vi "mqttTCPIPserver.vi"(0 "mqtt.lvclass":refnum<class "mqtt.lvclass">, 11 "error in (no error)":errorcluster) -> (4 "mqtt.lvclass 2":refnum<class "mqtt.lvclass">, 15 "error out":errorcluster)   [LabVIEW 2022 SP3, in "mqtt.lvclass"]
uses:
  mqtt.lvclass
  mqttTXqueue/mqttTXdataQueueFunction.ctl
  mqtt.lvclass/mqtt.ctl
  mqttTypedef/mqttRXdataCluster.ctl
  mqttTypedef/mqttFixedHeaderResponse.ctl
  mqttTypedef/mqttQOSlevel.ctl
  mqttTypedef/mqttMessageType.ctl
  mqttTXqueue/mqttRXsubscriptionEventFunction.ctl
  mqttTXqueue/mqttRXsubscriptionEventData.ctl
panel:
  out "rxCount":i32
  out "rxTelegram":u8[](array[numeric]) format="%02x"
  out "txError":errorcluster
  out "txTelegram":u8[](array[numeric]) format="%02x"
  out "payloadError":errorcluster
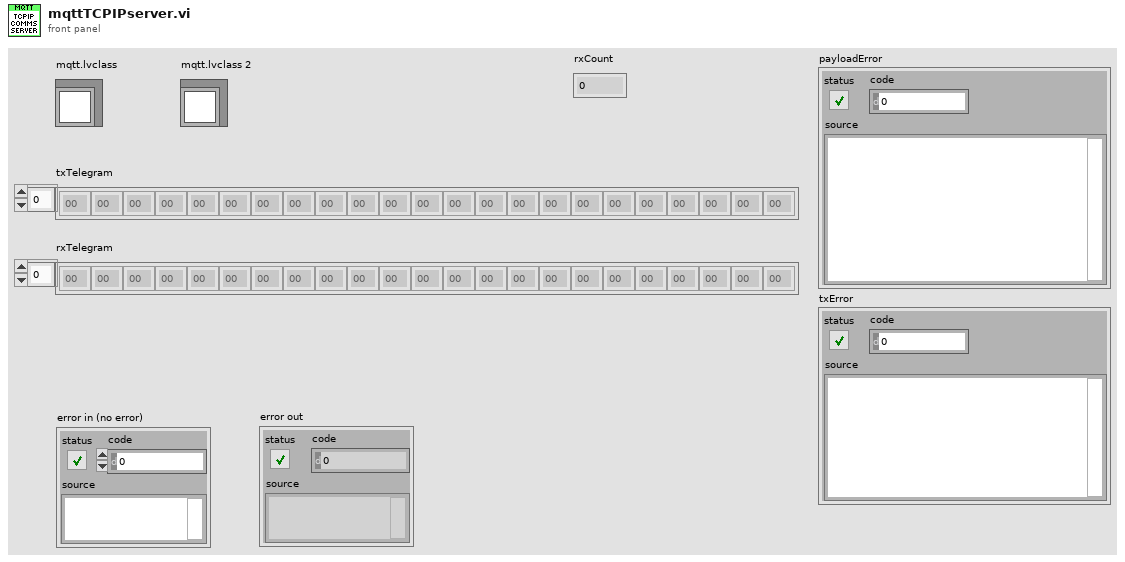
[diagram p1: front panel]
types:
  T1 = typedef "mqttTXdataQueueFunction.ctl" = enum16{"init", "deinit", "getQueue", "enqueue"}
  T2 = typedef "mqttRXdataCluster.ctl" = cluster{"fixedHdr":T3, "payload":u8[]}
  T3 = typedef "mqttFixedHeaderResponse.ctl" = cluster{"retain":bool, "qos":T4, "duplicate":bool, "response":T5}
  T4 = typedef "mqttQOSlevel.ctl" = enum8{"At most once", "At least once", "Exactly once", "Reserved"}
  T5 = typedef "mqttMessageType.ctl" = enum32{"Reserved", "CONNECT", "CONNACK", "PUBLISH", "PUBACK", "PUBREC", "PUBREL", "PUBCOMP", "SUBSCRIBE", "SUBACK", "UNSUBSCRIBE", "UNSUBACK", "PINGREQ", "PINGRESP", "DISCONNECT", "Reserved2"}
  T6 = typedef "mqttRXsubscriptionEventData.ctl" = cluster{"topic":string, "value":string, "messageID":u16}
  T7 = typedef "mqttRXsubscriptionEventFunction.ctl" = enum16{"init", "deinit", "getEventRef", "event"}
  T8 = typedef "mqttBroker.ctl" = cluster{"address":string, "port":u16, "connTimeout":i32, "writeTimeout":i32, "readTimeout":i32, "subTimeout":i32}
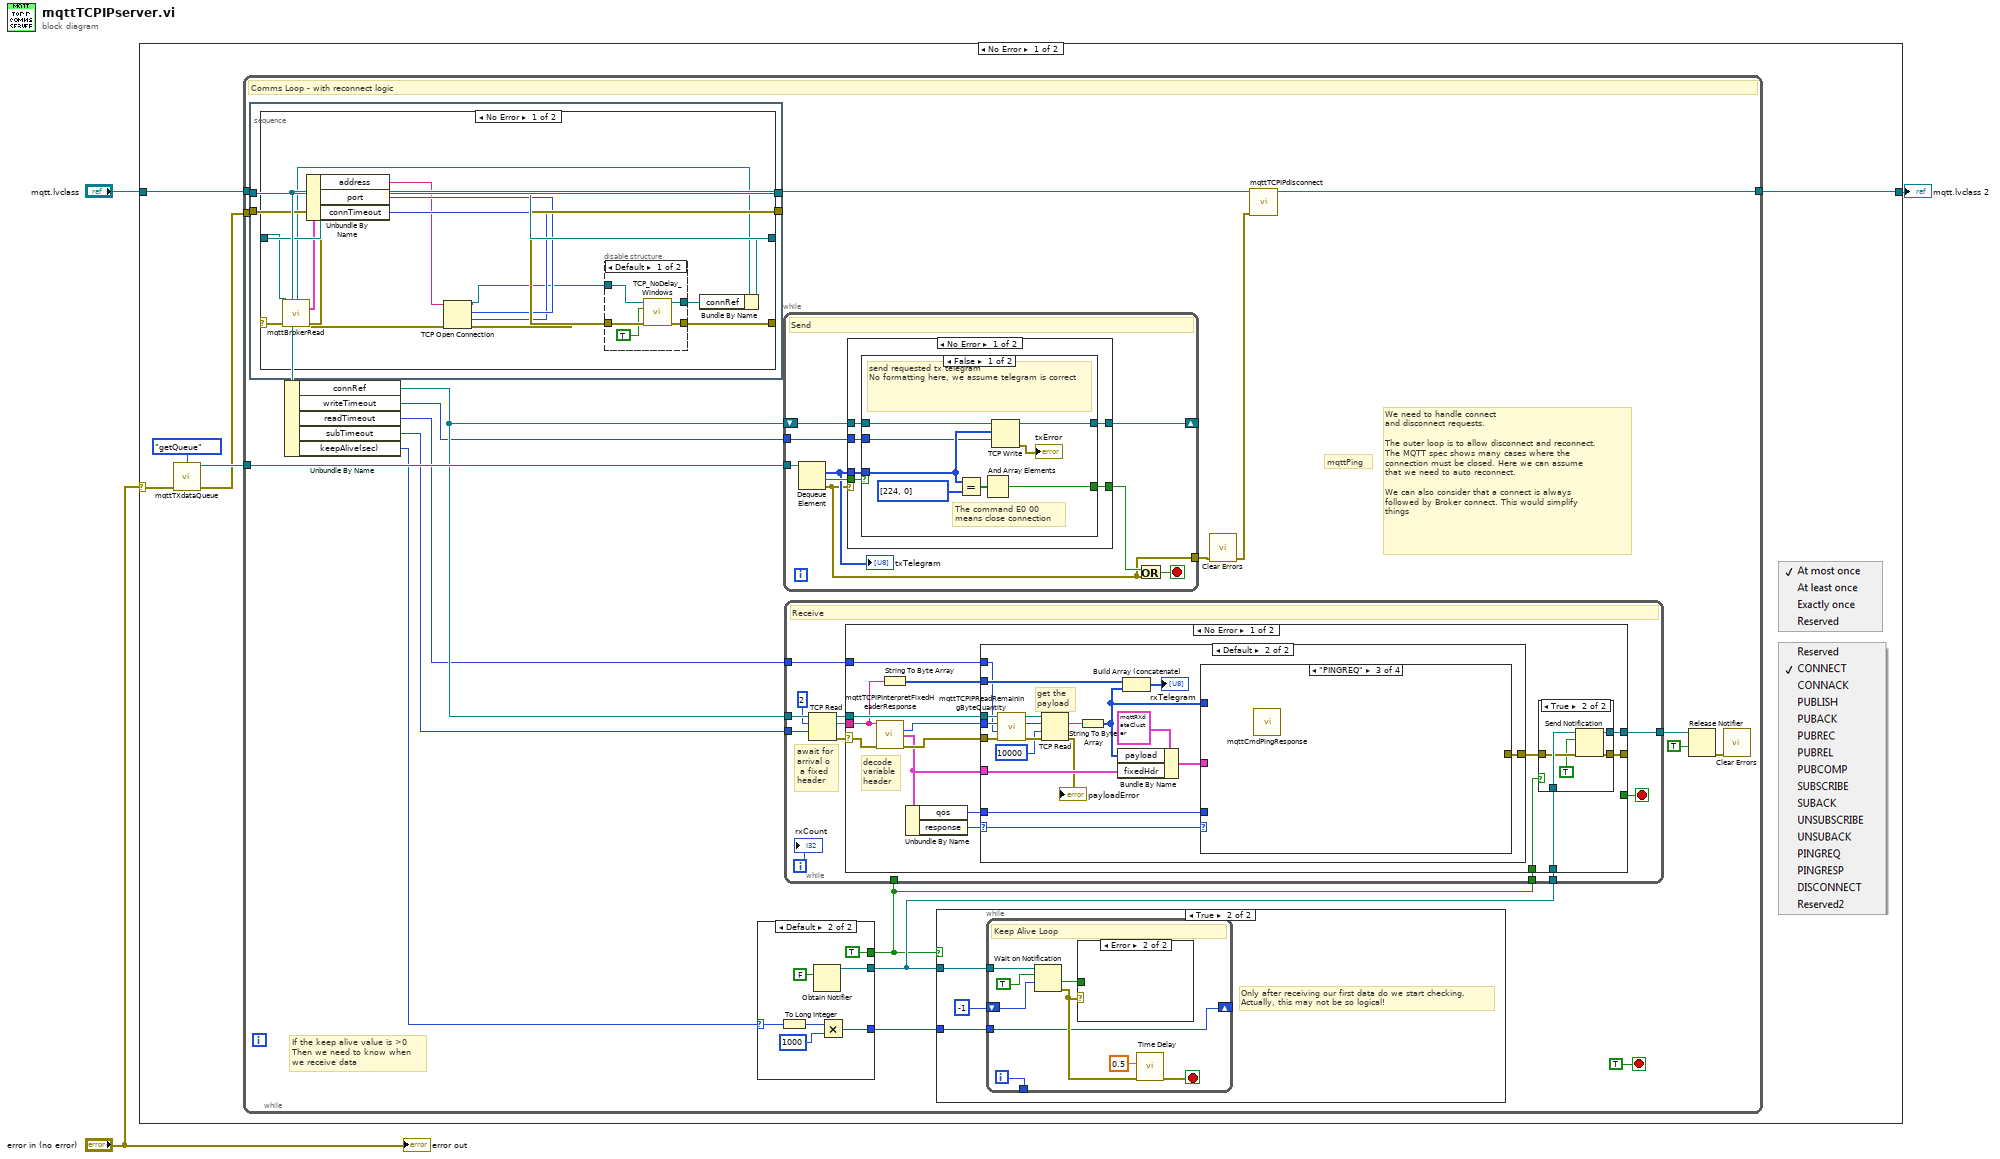
[diagram p0: block diagram]
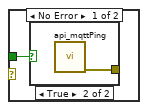
[diagram p5: hidden frame]
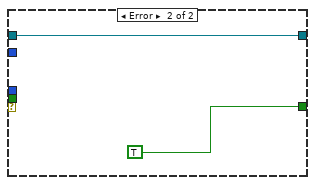
[diagram p9: hidden frame]
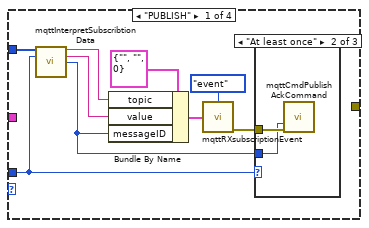
[diagram p12: hidden frame]
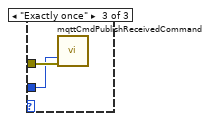
[diagram p14: hidden frame]
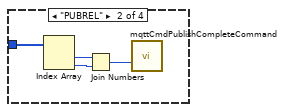
[diagram p15: hidden frame]
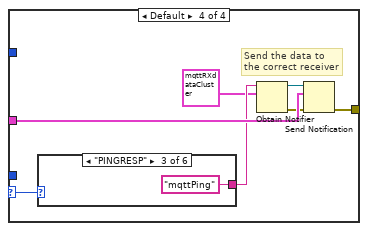
[diagram p16: hidden frame]
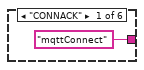
[diagram p17: hidden frame]
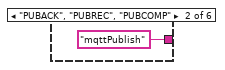
[diagram p18: hidden frame]
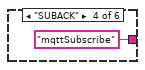
[diagram p19: hidden frame]
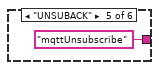
[diagram p20: hidden frame]
diagram:
  n1 = case shown="No Error" "error in (no error)" {
    selector: "error in (no error)" -> [w4 _]
    tunnel: "mqtt.lvclass" -> [w7 w189]
    tunnel: [w6 w189] -> w2
    frame No Error {
      n2 = call "mqttTXdataQueue.vi"("function"=mqttTXdataQueueFunction."getQueue", "error in (no error)"=w4) -> ("Queue out"=w9:refnum<queue>, "error out"=w5:errorcluster)  [unwired: 12 in]
      n3 = while {
        tunnel: w9 -> [w28]
        tunnel: w7 -> [w23]
        tunnel: [w21] -> w6
        tunnel: w5 -> [w22]
        stop <- TRUE stop-if-true
        # "If the keep alive value is >0\nThen we need to know when\nwe receive data"
        # "mqttPing"
        # "We need to handle connect\nand disconnect requests.\n\nThe outer loop is to allow disconnect and reconnect.\nThe MQTT spec shows many cases where the\nconnection must be closed. Here we can assume\nthat we need to auto reconnect.\n\nWe can also consider that a connect is always\nfollowed by Broker connect. This would simplify\nthings"
        # "Comms Loop - with reconnect logic"
        n4 = stacked-sequence {
          tunnel: w23 -> [w31]
          tunnel: [w32] -> w20
          tunnel: w22 -> [w29]
          tunnel: [w30] -> _
          frame #0 {
            n5 = case shown="No Error" w29 {
              selector: w29 -> [w43 w54]
              tunnel: [w44 w54] -> w30
              tunnel: [w36 w53] -> w32
              tunnel: w31 -> [w40 w53]
              frame No Error {
                n6 = call "mqttBrokerRead.vi"("mqtt in"=w40, "error in (no error)"=w43) -> ("mqtt out"=w38:refnum<class "mqtt.lvclass">, "broker"=w42:T8, "error out"=w34:errorcluster)  [unwired: 11 in]
                n7 = Unbundle By Name(w42) -> ("address"=w35:string, "port"=w41:u16, "connTimeout"=w39:i32)
                n8 = TCP Open Connection(address=w35, remote port or service name=w41, timeout ms (60000)=w39, error in (no error)=w34) -> (connection ID=w33:refnum<k5>, error out=w45:errorcluster)  [unwired: 1 in]
                n9 = disable-structure shown="Default" {
                  disable-tunnel: w45 -> [w50 w51]
                  disable-tunnel: [w49 w51] -> w44
                  disable-tunnel: [w47 w52] -> w37
                  disable-tunnel: w33 -> [w46 _]
                  frame condition #0 (active) {
                    n10 = call "TCP_NoDelay_Windows.vi"("error in (no error)"=w50, "TCP_NODELAY (true)"=TRUE, "connID"=w46) -> ("error out"=w49:errorcluster, "connID 2"=w47:refnum<k5>)  [unwired: 3 in]
                  }
                  frame condition #1 {
                  }
                }
                n11 = Bundle By Name(cluster=w38, "connRef"=w37) -> (w36:refnum<class "mqtt.lvclass">)
              }
              frame Error {
              }
            }
          }
        }
        n12 = Unbundle By Name(w20) -> ("connRef"=w26:refnum<k5>, "writeTimeout"=w19:i32, "readTimeout"=w18:i32, "subTimeout"=w17:i32, "keepAlive(sec)"=w11:u16)
        n13 = case shown="Default" w11 {
          selector: w11 -> [_ w70]
          tunnel: [_ w75] -> w16
          tunnel: [_ w71] -> w12
          tunnel: [_ TRUE] -> w10
          frame ..0 {
          }
          frame Default {
            n14 = To Long Integer(number=w70) -> (32bit integer=w73:i32)
            n15 = Obtain Notifier(notification data type=FALSE) -> (notifier out=w75:refnum<notifier>)  [unwired: 3 in, 2 out]
            n16 = Multiply(x=w73, y=1000) -> (x*y=w71:i32)
          }
        }
        n17 = while {
          tunnel: w28 -> [w84]
          shift-right: [w81] -> _
          shift-left: w26 -> [w82]
          tunnel: [w77] -> w25
          tunnel: w19 -> [w76]
          stop <- w80 stop-if-true
          # "Send"
          n18 = Dequeue Element(queue=w84) -> (element=w78:u8[], timed out?=w83:bool, error out=w77:errorcluster)  [unwired: 2 in, 1 out]
          "txTelegram" <- w78
          n19 = case shown="No Error" w77 {
            tunnel: w83 -> [w90 _]
            tunnel: w78 -> [w89 _]
            tunnel: w82 -> [w88 w101]
            tunnel: [w87 w101] -> w81
            tunnel: [w86 TRUE] -> w79
            tunnel: w76 -> [w85 _]
            frame No Error {
              n20 = case shown="False" w90 {
                tunnel: w89 -> [w96 _]
                tunnel: w88 -> [w98 w99]
                tunnel: [w97 w99] -> w87
                tunnel: [w93 _] -> w86
                tunnel: w85 -> [w91 _]
                frame False {
                  # "The command E0 00\nmeans close connection"
                  # "send requested tx telegram\nNo formatting here, we assume telegram is correct"
                  n21 = Equal?(x=w96, y=u8[] [224, 0] ("txTelegram 2")) -> (x = y?=w94:bool[])
                  n22 = And Array Elements(Boolean array=w94) -> (logical AND=w93:bool)
                  n23 = TCP Write(connection ID=w98, data in=w96, 9:w91) -> (connection ID out=w97:refnum<k5>, error out=→"txError":errorcluster)  [unwired: 1 in, 1 out]
                }
                frame True {
                  # "Queue Timed Out - do nothing.\nWe can later use this for the Keep Alive ping"
                }
              }
            }
            frame Error {
            }
          }
          n24 = Or(x=w79, y=w77) -> (x .or. y?=w80:bool)
        }
        n25 = while {
          tunnel: w26 -> [w113]
          tunnel: w18 -> [w106]
          tunnel: w17 -> [w105]
          tunnel: w16 -> [w104]
          tunnel: [w103] -> w15
          tunnel: w10 -> [w102]
          tunnel: w10 -> [_]
          i -> [w107]
          stop <- w108 stop-if-true
          # "await for\narrival o\n a fixed\nheader"
          # "Receive"
          n26 = TCP Read(connection ID=w113, bytes to read=2, 9:w105) -> (connection ID out=w112:refnum<k5>, data out=w109:string, error out=w111:errorcluster)  [unwired: 2 in]
          n27 = case shown="No Error" w111 {
            selector: w111 -> [w126 w188]
            tunnel: w112 -> [w127 _]
            tunnel: w109 -> [w122 _]
            tunnel: [_ w184] -> w108
            tunnel: w106 -> [w119 _]
            tunnel: w104 -> [w118 w183]
            tunnel: [w116 w183] -> w103
            tunnel: [w115 _] -> _
            tunnel: w102 -> [w114 _]
            frame No Error {
              # "decode\nvariable\nheader"
              n28 = call "mqttTCPIPInterpretFixedHeaderResponse.vi"("data in"=w122, "error in (no error)"=w126) -> ("remainingLengthByte1"=w128:u8, "output cluster"=w124:T3, "error out"=w125:errorcluster)  [unwired: 11 in]
              n29 = String To Byte Array(string=w122) -> (unsigned byte array=w121:u8[])
              n30 = Unbundle By Name(w124) -> ("qos"=w120:T4, "response"=w123:T5)
              n31 = case shown="Default" w123 {
                selector: w123 -> [_ w142]
                tunnel: w128 -> [_ w152]
                tunnel: w127 -> [_ w151]
                tunnel: w125 -> [_ w144]
                tunnel: w124 -> [_ w143]
                tunnel: w121 -> [_ w139]
                tunnel: w120 -> [_ w138]
                tunnel: w119 -> [_ w135]
                tunnel: [_ w134] -> w117
                frame "CONNECT", "SUBSCRIBE" {
                  # "The client should not receive these commands.\nI had some problems with these commands being received\nand it appears this was a broker issue. However, to ignore\nmessages that we should not receive is no bad thing."
                }
                frame Default {
                  # "get the\npayload"
                  n32 = call "mqttTCPIPReadRemainingByteQuantity.vi"("error in (no error)"=w144, "readTimeout ms (2000)"=w135, "remainingLengthByte1"=w152, "connRef in"=w151) -> ("error out"=w149:errorcluster, "remainingLength"=w148:i32, "connRef out"=w150:refnum<k5>)  [unwired: 5 in]
                  n33 = TCP Read(connection ID=w150, bytes to read=w148, error in (no error)=w149, 9:10000 ("timeout ms (25000)")) -> (data out=w146:string, error out=→"payloadError":errorcluster)  [unwired: 1 in, 1 out]
                  n34 = String To Byte Array(string=w146) -> (unsigned byte array=w136:u8[])
                  n35 = Bundle By Name(cluster=T2 {"fixedHdr"={"retain"=FALSE, "qos"=enum."At most once", "duplicate"=FALSE, "response"=enum."Reserved"}, "payload"=[]} ("output cluster"), "payload"=w136, "fixedHdr"=w143) -> (w140:T2)
                  n36 = Build Array (concatenate)(w139, w136) -> (→"rxTelegram":u8[])
                  n37 = case shown="\"PINGREQ\"" w142 {
                    selector: w142 -> [_ _ _ w176]
                    tunnel: w140 -> [_ _ _ w175]
                    tunnel: w138 -> [w154 _ _ _]
                    tunnel: w136 -> [w158 w169 _ _]
                    tunnel: [_ _ _ w170] -> w134
                    frame "PUBLISH" {
                      n38 = call "mqttInterpretSubscribtionData.vi"("rxTelegram in"=w158, "qos"=w154) -> ("topic"=w157:string, "value"=w156:string, "messageID"=w153:u16)  [unwired: 10 in, 1 out]
                      n39 = Bundle By Name(cluster=T6 {"topic"="", "value"="", "messageID"=0} ("data"), "topic"=w157, "value"=w156, "messageID"=w153) -> (w159:T6)
                      n40 = call "mqttRXsubscriptionEvent.vi"("function"=mqttRXsubscriptionEventFunction."event", "data"=w159) -> ("error out"=w155:errorcluster)  [unwired: 12 in, 1 out]
                      n41 = case shown="\"At least once\"" w154 {
                        tunnel: w155 -> [_ w163 w165]
                        tunnel: w153 -> [_ w162 w164]
                        frame Default {
                        }
                        frame "At least once" {
                          n42 = call "mqttCmdPublishAckCommand.vi"("messageID"=w162, "error in (no error)"=w163) -> ()  [unwired: 13 in, 1 out]
                        }
                        frame "Exactly once" {
                          n43 = call "mqttCmdPublishReceivedCommand.vi"("messageID"=w164, "error in (no error)"=w165) -> ()  [unwired: 13 in, 1 out]
                        }
                      }
                    }
                    frame "PUBREL" {
                      n44 = Index Array(array=w169) -> (element #1=w168:u8, element #2=w167:u8)  [unwired: 2 in]
                      n45 = Join Numbers(hi=w168, lo=w167) -> ((hi.lo)=w166:u16)
                      n46 = call "mqttCmdPublishCompleteCommand.vi"("messageID"=w166) -> ()  [unwired: 14 in, 1 out]
                    }
                    frame "PINGREQ" {
                      n47 = call "mqttCmdPingResponse.vi"() -> ()  [unwired: 15 in, 1 out]
                    }
                    frame Default {
                      # "Send the data to\nthe correct receiver"
                      n48 = case shown="\"PINGRESP\"" w176 {
                        tunnel: ["mqttConnect" ("name (unnamed)") "mqttPublish" ("name (unnamed)") "mqttPing" ("name (unnamed)") "mqttSubscribe" ("name (unnamed)") "mqttUnsubscribe" ("name (unnamed)") "mqttError" ("name (unnamed)")] -> w174
                        frame "CONNACK" {
                        }
                        frame "PUBACK", "PUBREC", "PUBCOMP" {
                        }
                        frame "PINGRESP" {
                        }
                        frame "SUBACK" {
                        }
                        frame "UNSUBACK" {
                        }
                        frame Default {
                        }
                      }
                      n49 = Obtain Notifier(name (unnamed)=w174, notification data type=T2 {"fixedHdr"={"retain"=FALSE, "qos"=enum."At most once", "duplicate"=FALSE, "response"=enum."Reserved"}, "payload"=[]} ("output cluster")) -> (notifier out=w173:refnum<notifier>, error out=w171:errorcluster)  [unwired: 2 in, 1 out]
                      n50 = Send Notification(notification=w175, notifier=w173, error in (no error)=w171) -> (error out=w170:errorcluster)  [unwired: 1 out]
                    }
                  }
                }
              }
              n51 = case shown="True" w114 {
                tunnel: w118 -> [_ w133]
                tunnel: w117 -> [_ w132]
                tunnel: [_ w130] -> w116
                tunnel: [_ w129] -> w115
                frame False {
                }
                frame True {
                  n52 = Send Notification(notification=TRUE, notifier=w133, error in (no error)=w132) -> (notifier out=w130:refnum<notifier>, error out=w129:errorcluster)
                }
              }
            }
            frame Error {
              # "Find what the code is for timeout\nIf we did not timeout, we had an unhandled error and so stop"
              n53 = Unbundle By Name(w188) -> ("code"=w187:i32)
              n54 = Not Equal?(x=w187, y=i32[] [56, 59]) -> (x != y?=w185:bool[])
              n55 = Or Array Elements(Boolean array=w185) -> (logical OR=w184:bool)
            }
          }
          "rxCount" <- w107
        }
        n56 = case shown="True" w10 {
          tunnel: w16 -> [_ w57]
          tunnel: w12 -> [_ w56]
          frame False {
          }
          frame True {
            # "Only after receiving our first data do we start checking.\nActually, this may not be so logical!"
            n57 = while {
              tunnel: w57 -> [w66]
              tunnel: [w61] -> _
              shift-right: [w58] -> _
              shift-left: -1 -> [w65]
              tunnel: w56 -> [w58]
              i -> [w61]
              stop <- w62 stop-if-true
              # "Keep Alive Loop"
              n58 = Wait on Notification(notifier=w66, ignore previous (F)=TRUE, timeout in ms (-1)=w65) -> (timed out?=w64:bool, error out=w59:errorcluster)  [unwired: 1 in, 2 out]
              n59 = case shown="Error" w59 {
                tunnel: w64 -> [w67 _]
                frame No Error {
                  n60 = case shown="True" w67 {
                    tunnel: [_ w68] -> _
                    frame False {
                    }
                    frame True {
                      n61 = call "api_mqttPing.vi"() -> ("error out"=w68:errorcluster)  [unwired: 14 in, 1 out]
                    }
                  }
                }
                frame Error {
                }
              }
              n62 = call "Time Delay"("error in (no error)"=w59, "Delay Time (s)"=0.5) -> ("error out"=w62:errorcluster)  [unwired: 9 in]
            }
          }
        }
        n63 = call <vilib>:"Clear Errors.vi"("error in (no error)"=w25) -> ("error out"=w24:errorcluster)  [unwired: 5 in, 1 out]
        n64 = call "mqttTCPIPdisconnect.vi"("mqtt in"=w20, "error in (no error)"=w24) -> ("mqtt out"=w21:refnum<class "mqtt.lvclass">)  [unwired: 12 in, 1 out]
        n65 = Release Notifier(notifier=w15, force destroy? (F)=TRUE) -> (error out=w13:errorcluster)  [unwired: 1 in, 2 out]
        n66 = call <vilib>:"Clear Errors.vi"("error in (no error)"=w13) -> ()  [unwired: 5 in, 2 out]
      }
    }
    frame Error {
    }
  }
  "mqtt.lvclass 2" <- w2
  "error out" <- "error in (no error)"
